vi "Build StoryArc Report.vi"() -> ()   [LabVIEW 2024]
uses:
  manager_daemon/type_defs/sub-map--map.ctl
  manager_daemon/type_defs/SubData--cluster.ctl
  manager_daemon/type_defs/IssueData--clustrer.ctl
  manager_daemon/manager_daemon.lvclass
panel:
  in  "Boolean":bool
  out "reversed array":T1(array[cluster]) {"Array"."cover_date" format="%<%x>T"}
  out "data":T2
  out "error out":errorcluster
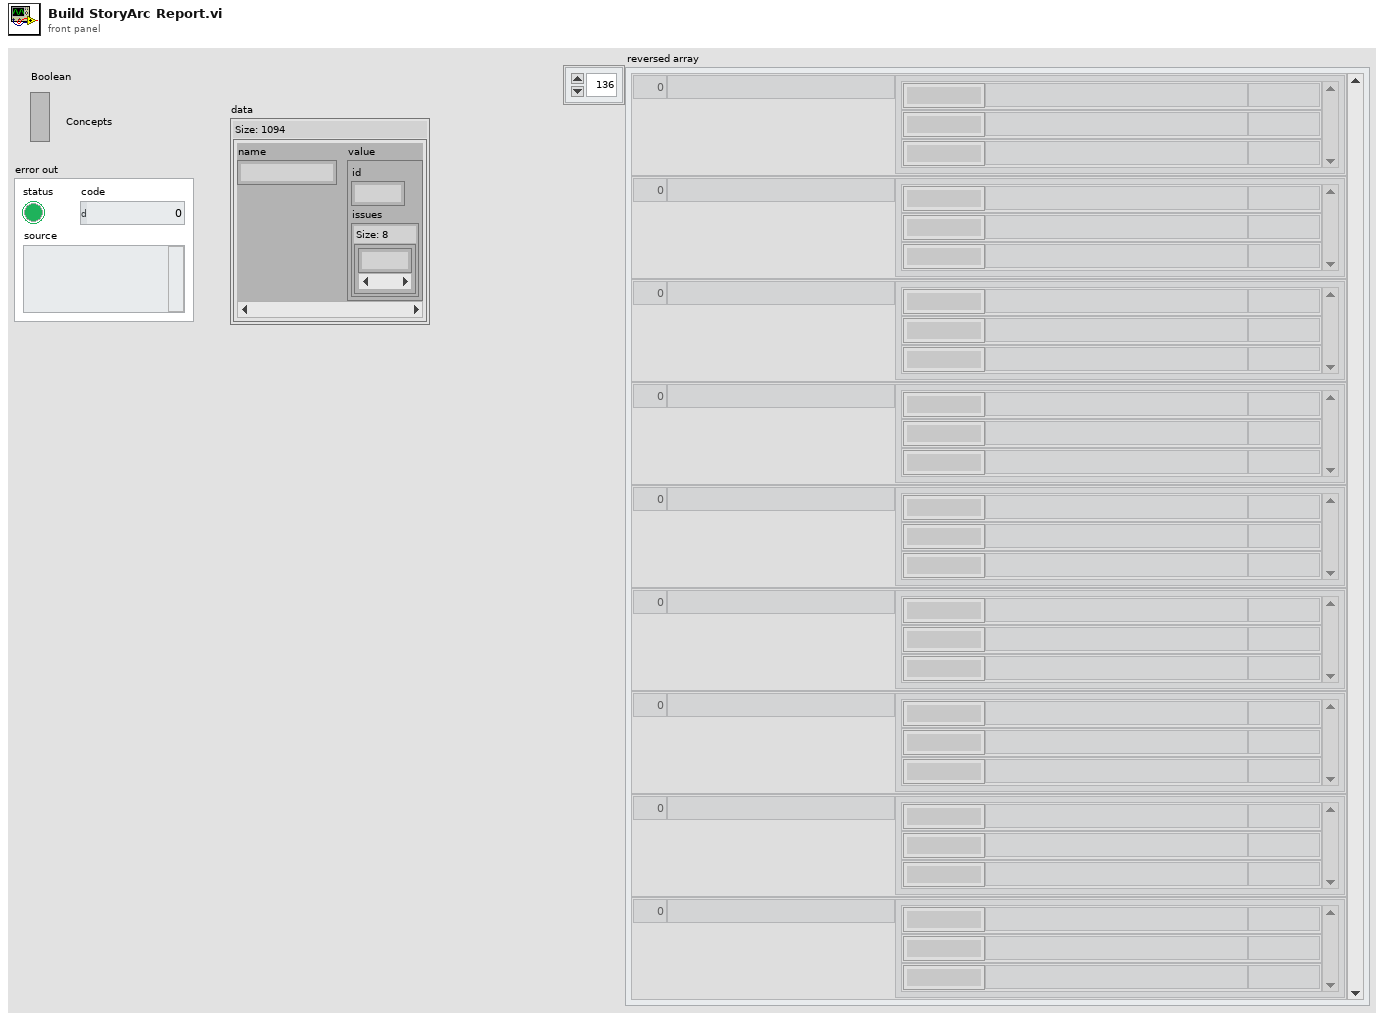
[diagram p1: front panel]
types:
  T1 = cluster{"Numeric":i32, "name":string, "Array":cluster{"cover_date":timestamp, "sortable_name":string, "sortable_name":string}[]}[]
  T2 = typedef "manager_daemon.lvclass/sub-map--map.ctl" = map{string, T3}
  T3 = typedef "manager_daemon.lvclass/SubData--cluster.ctl" = cluster{"id":i32, "issues":set{i32}}
  T4 = typedef "manager_daemon.lvclass/IssueData--clustrer.ctl" = cluster{"cover_date":timestamp, "cv_id":string, "name":string, "sortable_name":string, "issue_number":string, "deck":string, "description":string, "id":i32, "store_date":timestamp, "date_last_updated":timestamp, "site_detail_url":string, "cover_url":string, "source_path":path}
  T5 = cluster{"cover_date":timestamp, "sortable_name":string, "sortable_name":string}
  T6 = cluster{"cover_date":timestamp, "sortable_name":string, "sortable_name":string}[]
  T7 = cluster{i32, "name":string, cluster{"cover_date":timestamp, "sortable_name":string, "sortable_name":string}[]}
  T8 = cluster{i32, "name":string, cluster{"cover_date":timestamp, "sortable_name":string, "sortable_name":string}[]}[]
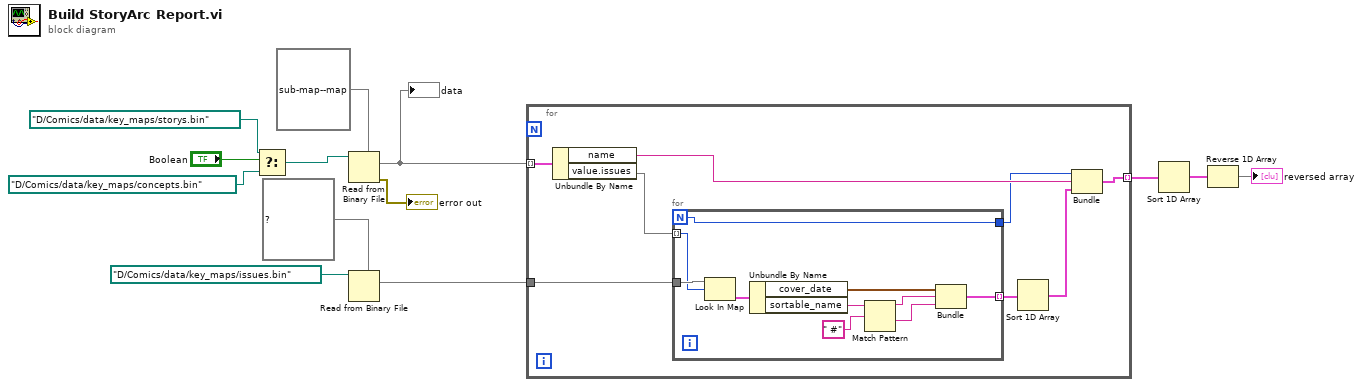
[diagram p0: block diagram]
diagram:
  n1 = Select(t=path "D:/Comics/data/key_maps/storys.bin" ("file (use dialog)"), s="Boolean", f=path "D:/Comics/data/key_maps/concepts.bin" ("file (use dialog)")) -> (s? t:f=w2:path)
  n2 = Read from Binary File(5:T2 {} ("story map"), 11:w2) -> (0:→"error out":errorcluster, 2:w11:T2)  [unwired: 4 in, 2 out]
  "data" <- w11
  n3 = Read from Binary File(5:map{i32, T4} {} ("issue map"), 11:path "D:/Comics/data/key_maps/issues.bin" ("file (use dialog)")) -> (2:w7:map{i32, T4})  [unwired: 4 in, 3 out]
  n4 = for {
    tunnel: w11 -> [w21] mode=indexing
    tunnel: [w19] -> w6 mode=indexing
    tunnel: w7 -> [w17]
    n5 = Unbundle By Name(w21) -> ("name"=w20:string, "value.issues"=w18:set{i32})
    n6 = for {
      N -> [w22]
      tunnel: w18 -> [w30] mode=indexing
      tunnel: w17 -> [w31]
      tunnel: [w23] -> w15 mode=indexing
      tunnel: [w22] -> w16
      n7 = Look In Map(map=w31, key=w30) -> (value=w29:T4)  [unwired: 1 in, 1 out]
      n8 = Unbundle By Name(w29) -> ("cover_date"=w26:timestamp, "sortable_name"=w28:string)
      n9 = Match Pattern(string=w28, regular expression=" #") -> (before substring=w25:string, after substring=w24:string)  [unwired: 1 in, 2 out]
      n10 = Bundle("cover_date"=w26, "sortable_name"=w25, "sortable_name"=w24) -> (w23:T5)  [unwired: 1 in]
    }
    n11 = Sort 1D Array(array=w15) -> (sorted array=w14:T6)
    n12 = Bundle(w16, "name"=w20, w14) -> (w19:T7)  [unwired: 1 in]
  }
  n13 = Sort 1D Array(array=w6) -> (sorted array=w10:T8)
  n14 = Reverse 1D Array(array=w10) -> (reversed array=→"reversed array":T8)
